vi "Cache.Result.NextToExport.vi"(8 "error in (no error)":errorcluster, 11 "SystemIdx":i32) -> (0 "error out":errorcluster, 3 "files to export":path[](array[path]))   [LabVIEW 2016]
uses:
  Global/ApplicationGlobal.vi
panel:
  out "delay":u32
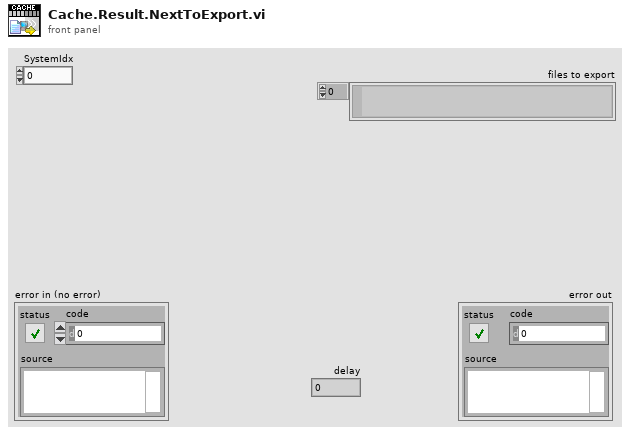
[diagram p1: front panel]
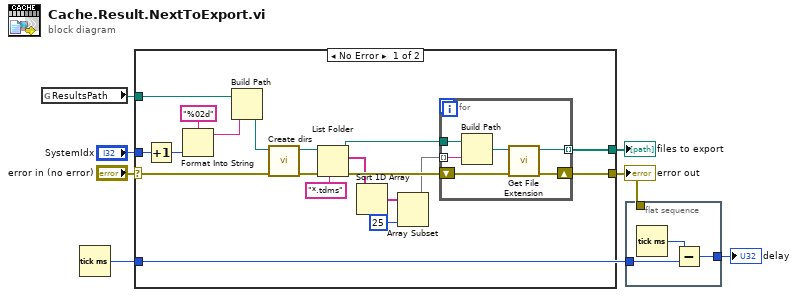
[diagram p0: block diagram]
diagram:
  n1 = global read "ApplicationGlobal.vi" "ResultsPath"() -> (w6:path)
  n2 = Tick Count (ms)() -> (millisecond timer value=w3:u32)
  n3 = case shown="No Error" "error in (no error)" {
    selector: "error in (no error)" -> [w10 w31]
    tunnel: [w22 w31] -> w4
    tunnel: w6 -> [w19 _]
    tunnel: [w21 _] -> w1
    tunnel: "SystemIdx" -> [w11 _]
    tunnel: w3 -> [_ _]
    frame No Error {
      n4 = Increment(x=w11) -> (x+1=w16:i32)
      n5 = Format Into String(format string="%02d", w16) -> (resulting string=w18:string)  [unwired: 2 in, 1 out]
      n6 = Build Path(base path=w19, name or relative path=w18) -> (appended path=w8:path)
      n7 = call "Create dirs.vi"("error in (no error)"=w10, "deepest dir"=w8) -> ("error"=w9:errorcluster)  [unwired: 9 out]
      n8 = List Folder(path=w8, pattern="*.tdms", error in=w9) -> (path out=w23:path, filenames=w15:string[], error out=w24:errorcluster)  [unwired: 1 in, 1 out]
      n9 = Sort 1D Array(array=w15) -> (sorted array=w13:string[])
      n10 = Array Subset(array=w13, length=25) -> (w12:string[])  [unwired: 1 in]
      n11 = for {
        tunnel: w12 -> [w29] mode=indexing
        tunnel: w23 -> [w30]
        shift-right: [w26] -> w22
        shift-left: w24 -> [w28]
        tunnel: [w25] -> w21 mode=indexing
        # "through all files"
        n12 = Build Path(base path=w30, name or relative path=w29) -> (appended path=w27:path)
        n13 = call <vilib>:"Get File Extension.vi"("error in (no error)"=w28, "file"=w27) -> ("error out"=w26:errorcluster, "dup file"=w25:path)  [unwired: 5 in, 3 out]
      }
    }
    frame Error {
    }
  }
  "error out" <- w4
  "files to export" <- w1
  n14 = flat-sequence {
    tunnel: w4 -> [_]
    tunnel: w3 -> [w34]
    tunnel: [w32] -> w2
    frame #0 {
      n15 = Tick Count (ms)() -> (millisecond timer value=w33:u32)
      n16 = Subtract(x=w33, y=w34) -> (x-y=w32:u32)
    }
  }
  "delay" <- w2
